vi "Parse Response JSON.vi"(8 "error in (no error)":errorcluster, 10 "Response JSON":string, 11 "RGetInputMute in":refnum<class "RGetInputMute.lvclass">) -> (0 "error out":errorcluster, 3 "RGetInputMute out":refnum<class "RGetInputMute.lvclass">)   [LabVIEW 2020, in "obs-websocket.lvlib" / "RGetInputMute.lvclass"]
uses:
  RGetInputMute.lvclass
  RGetInputMute.lvclass/RGetInputMute.ctl
  04e1b71b-5261-43cc-b8e6-198a401c5565.vi
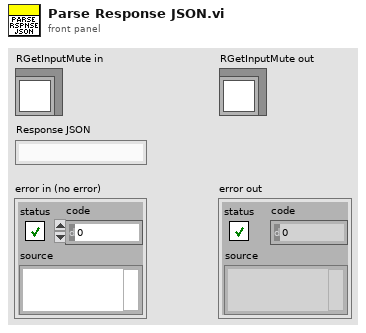
[diagram p1: front panel]
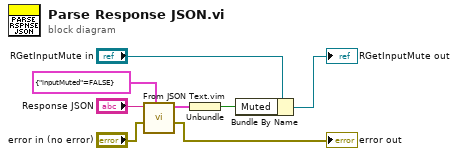
[diagram p0: block diagram]
diagram:
  n1 = call "From JSON Text.vim"("Data Type and Default Value"=cluster{"inputMuted":bool} {"inputMuted"=FALSE}, "error in (no error)"="error in (no error)", "JSON"="Response JSON") -> ("error out"=→"error out":errorcluster, "Data out"=w4:cluster{"inputMuted":bool})  [unwired: 7 in]
  n2 = Unbundle(w4) -> ("inputMuted"=w3:bool)
  n3 = Bundle By Name(cluster="RGetInputMute in", "Muted"=w3) -> (→"RGetInputMute out":refnum<class "RGetInputMute.lvclass">)
